vi "JKISM++ Example - Caller is NOT JKISM.vi"() -> ()   [LabVIEW 2014]
uses:
  user.lib/_NEVSTOP/JKI State Machine++/_Support/JKISMQ/_Create Data Queue.vi
  user.lib/_NEVSTOP/JKI State Machine++/_Support/JKISMQ/_JKISMQFGV.vi
  user.lib/_NEVSTOP/JKI State Machine++/JKI State Machine++.lvlib
panel:
  in  "UI: Front Panel State >> Close":bool
  in  "UI: Front Panel State >> Open":bool
  in  "API: Get Level":bool
  in  "Target Module":string(combo)="SubModule0"
  in  "Level":dbl min=0.0 max=1.0 step=0.1
  out "State History of Main":string
  in  "API: Stop":bool
  in  "API: Start":bool
  in  "Unregister Status Change":bool
  in  "Register Status Change":bool
  out "error":errorcluster
  in  "Stop Module":bool
  in  "Start Module":bool
  out "Exist?":bool
  # "Start/Stop Module"
  # "asdfasf"
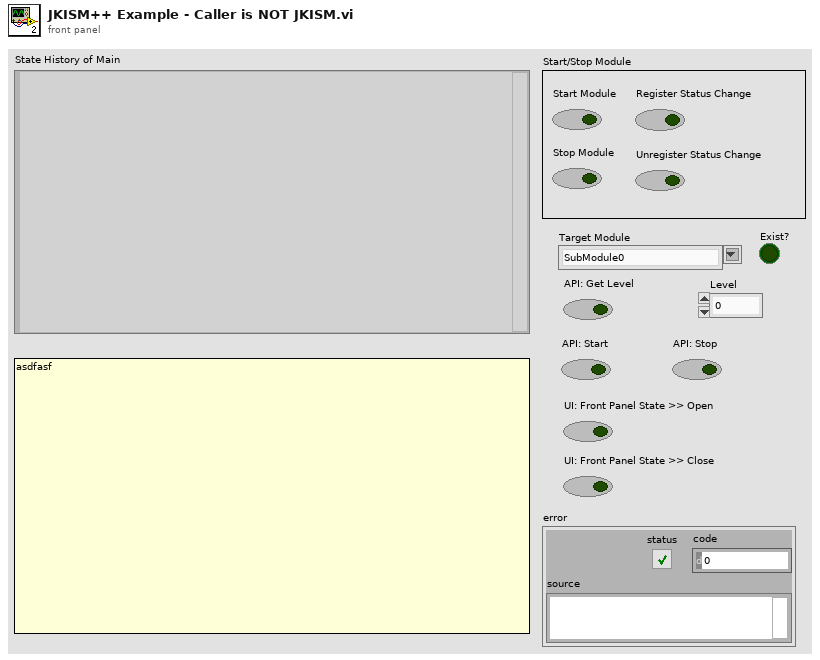
[diagram p1: front panel]
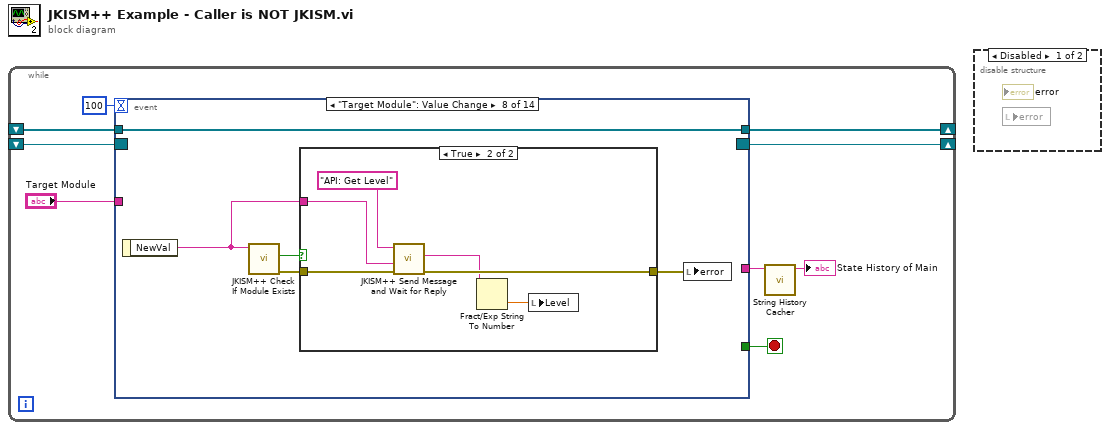
[diagram p0: block diagram]
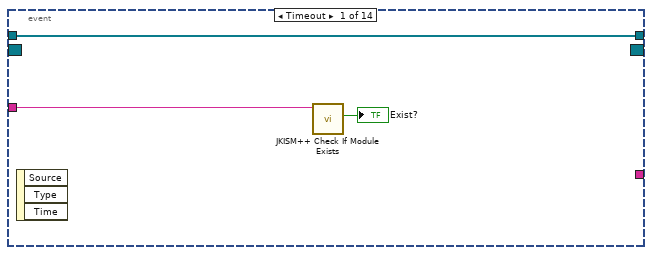
[diagram p3: hidden frame]
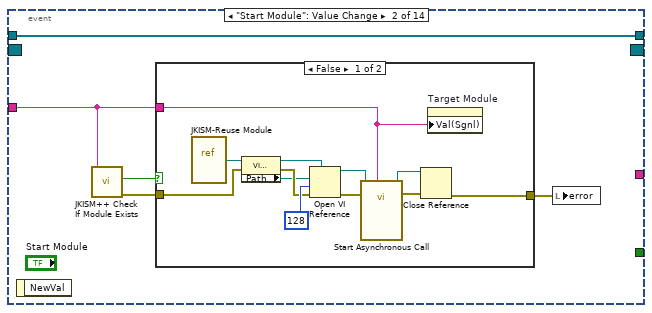
[diagram p4: hidden frame]
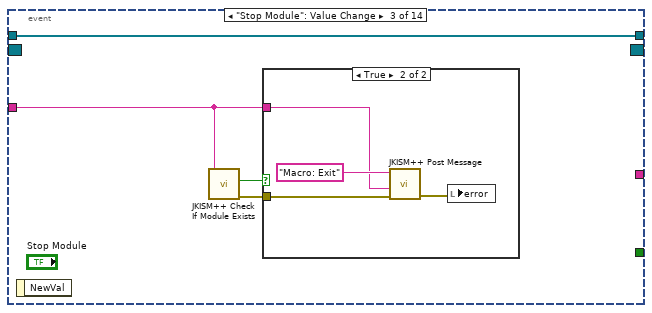
[diagram p6: hidden frame]
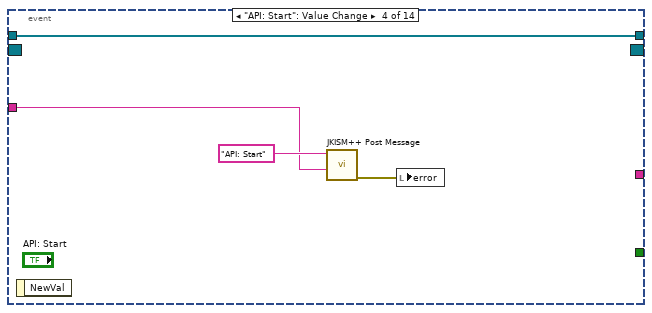
[diagram p8: hidden frame]
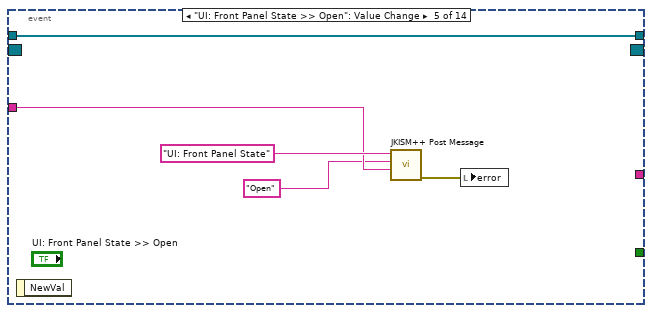
[diagram p9: hidden frame]
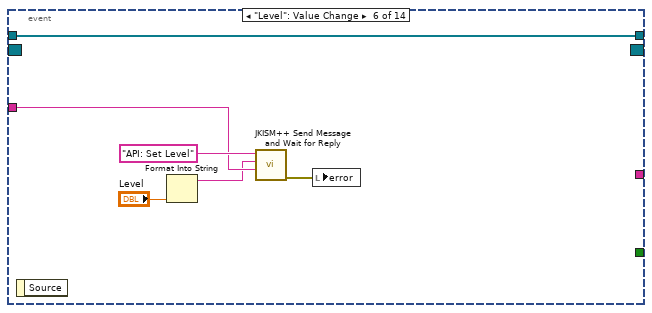
[diagram p10: hidden frame]
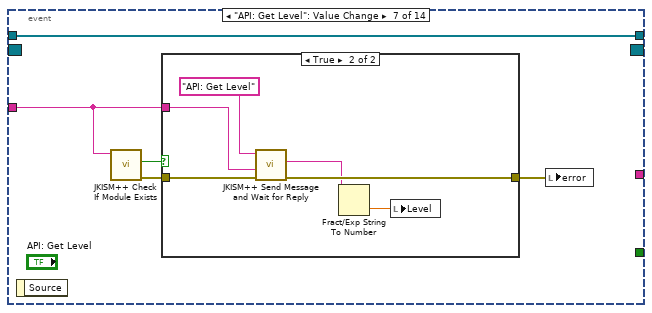
[diagram p11: hidden frame]
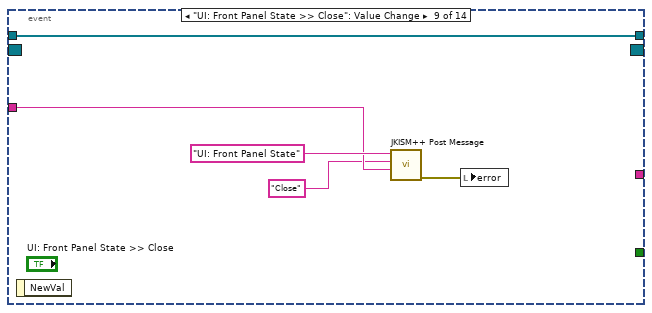
[diagram p14: hidden frame]
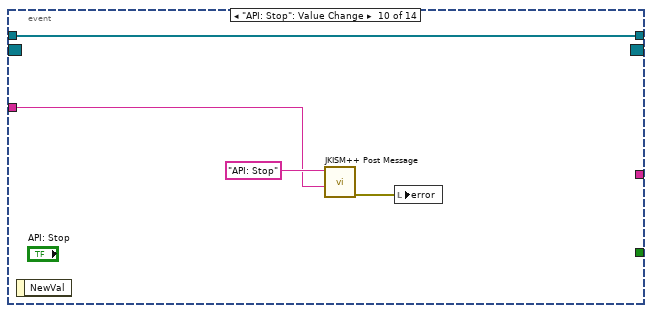
[diagram p15: hidden frame]
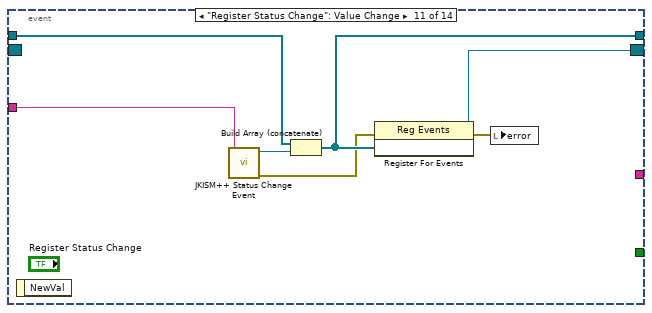
[diagram p16: hidden frame]
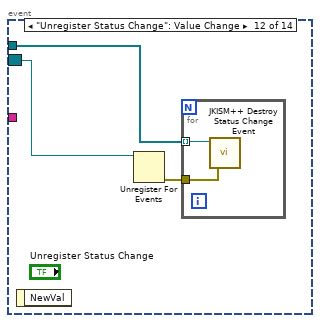
[diagram p17: hidden frame]
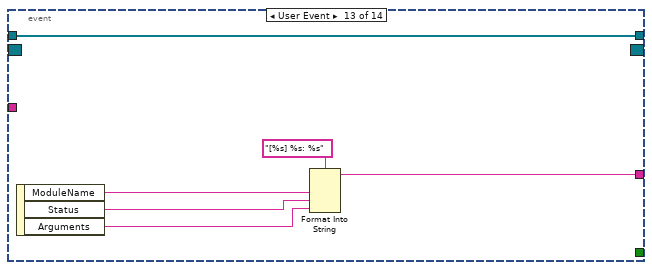
[diagram p18: hidden frame]
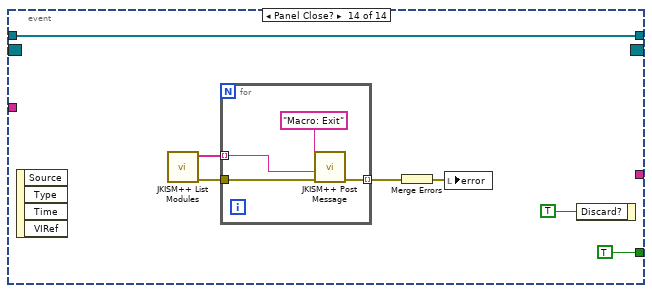
[diagram p19: hidden frame]
diagram:
  n1 = while {
    shift-right: [w7] -> _
    shift-left: _ -> [w6]
    shift-right: [w5] -> _
    shift-left: _ -> [w4]
    stop <- w9 stop-if-true
    n2 = event shown="[7] \"Target Module\": Value Change" {
      selector: w6 -> [_ _ _ _ _ _ _ _ _ _ _ w96 _ _]
      dyn-events: [_ _ _ _ _ _ _ _ _ _ w93 _ _ _] -> w7
      timeout: 100 -> [_ _ _ _ _ _ _ _ _ _ _ _ _ _]
      tunnel: [_ _ _ _ _ _ _ _ _ _ _ _ _ TRUE ("Discard?")] -> w9
      tunnel: [w12 w17 w34 w40 w45 w51 w57 w69 w80 w84 w92 _ w99 w109] -> w5
      tunnel: w4 -> [w12 w17 w34 w40 w45 w51 w57 w69 w80 w84 w90 w94 w99 w109]
      tunnel: [_ _ _ _ _ _ _ _ _ _ _ _ w100 _] -> w2
      tunnel: "Target Module" -> [w10 w13 w31 w39 w44 w50 w56 _ w79 w83 w89 _ _ _]
      event Timeout {
        n3 = event-data() -> ()  [unwired: 1 in, 3 out]
        n4 = call "JKISM++ Check If Module Exists.vi"("JKISM Name"=w10) -> ("Exist?"=→"Exist?":bool)  [unwired: 8 in, 2 out]
      }
      event "Start Module": Value Change {
        n5 = event-data() -> ()  [unwired: 1 in, 1 out]
        n6 = call "JKISM++ Check If Module Exists.vi"("JKISM Name"=w13) -> ("Error out"=w15:errorcluster, "Exist?"=w16:bool)  [unwired: 8 in, 1 out]
        n7 = case shown="False" w16 {
          tunnel: w15 -> [w20 w30]
          tunnel: [w19 w30] -> w14
          tunnel: w13 -> [w18 _]
          frame False {
            n8 = vi-ref "JKISM-Reuse Module.vi"() -> (w22:refnum<vi>)
            n9 = property class="VI (strict)"(reference=w22, error in=w20) -> (reference out=w26:refnum<vi>, error out=w24:errorcluster, "Path"=w23:path)
            n10 = Open VI Reference(type specifier VI Refnum (for type only)=w26, vi path=w23, options=128, error in (no error)=w24) -> (vi reference=w25:refnum<vi>, error out=w21:errorcluster)  [unwired: 2 in]
            n11 = call-by-ref "Start Asynchronous Call"(reference=w25, error in=w21, "Name(\"\" to use uuid)"=w18) -> (reference out=w28:refnum<vi>, error out=w27:errorcluster)  [unwired: 11 in]
            n12 = Close Reference(reference=w28, error in (no error)=w27) -> (error out=w19:errorcluster)
            n13 = property on="Target Module" class="CmbBox"("Val(Sgnl)"=w18) -> ()  [unwired: 2 in, 2 out]
          }
          frame True {
          }
        }
        n14 = local write "error"(w14) -> ()
      }
      event "Stop Module": Value Change {
        n15 = event-data() -> ()  [unwired: 1 in, 1 out]
        n16 = call "JKISM++ Check If Module Exists.vi"("JKISM Name"=w31) -> ("Error out"=w32:errorcluster, "Exist?"=w33:bool)  [unwired: 8 in, 1 out]
        n17 = case shown="True" w33 {
          tunnel: w32 -> [_ w36]
          tunnel: w31 -> [_ w35]
          frame False {
          }
          frame True {
            n18 = call "JKISM++ Post Message.vi"("Error In (no error)"=w36, "Target Module"=w35, "State"="Macro: Exit" ("States")) -> ("error out"=w37:errorcluster)  [unwired: 8 in]
            n19 = local write "error"(w37) -> ()
          }
        }
      }
      event "API: Start": Value Change {
        n20 = event-data() -> ()  [unwired: 1 in, 1 out]
        n21 = call "JKISM++ Post Message.vi"("Target Module"=w39, "State"="API: Start") -> ("error out"=w41:errorcluster)  [unwired: 9 in]
        n22 = local write "error"(w41) -> ()
      }
      event "UI: Front Panel State >> Open": Value Change {
        n23 = event-data() -> ()  [unwired: 1 in, 1 out]
        n24 = call "JKISM++ Post Message.vi"("Target Module"=w44, "Arguments (\"\")"="Open" ("Arguments (\"\")"), "State"="UI: Front Panel State") -> ("error out"=w46:errorcluster)  [unwired: 8 in]
        n25 = local write "error"(w46) -> ()
      }
      event "Level": Value Change {
        n26 = event-data() -> ()  [unwired: 1 in, 1 out]
        n27 = Format Into String("Level") -> (resulting string=w48:string)  [unwired: 3 in, 1 out]
        n28 = call "JKISM++ Send Message and Wait for Reply.vi"("Target Module"=w50, "Arguments (\"\")"=w48, "State"="API: Set Level") -> ("error out"=w52:errorcluster)  [unwired: 7 in, 1 out]
        n29 = local write "error"(w52) -> ()
      }
      event "API: Get Level": Value Change {
        n30 = event-data() -> ()  [unwired: 1 in, 1 out]
        n31 = call "JKISM++ Check If Module Exists.vi"("JKISM Name"=w56) -> ("Error out"=w55:errorcluster, "Exist?"=w54:bool)  [unwired: 8 in, 1 out]
        n32 = case shown="True" w54 {
          tunnel: [w59 w64] -> w58
          tunnel: w56 -> [_ w61]
          tunnel: w55 -> [w59 w60]
          frame False {
          }
          frame True {
            n33 = call "JKISM++ Send Message and Wait for Reply.vi"("Error In (no error)"=w60, "Target Module"=w61, "State"="API: Get Level") -> ("error out"=w64:errorcluster, "Arguments"=w62:string)  [unwired: 7 in]
            n34 = Fract/Exp String To Number(string=w62) -> (number=w63:dbl)  [unwired: 3 in, 1 out]
            n35 = local write "Level"(w63) -> ()
          }
        }
        n36 = local write "error"(w58) -> ()
      }
      event "Target Module": Value Change {
        n37 = event-data() -> ("NewVal"=w66:string)  [unwired: 1 in]
        n38 = call "JKISM++ Check If Module Exists.vi"("JKISM Name"=w66) -> ("Error out"=w68:errorcluster, "Exist?"=w67:bool)  [unwired: 8 in, 1 out]
        n39 = case shown="True" w67 {
          tunnel: [w71 w76] -> w70
          tunnel: w66 -> [_ w73]
          tunnel: w68 -> [w71 w72]
          frame False {
          }
          frame True {
            n40 = call "JKISM++ Send Message and Wait for Reply.vi"("Error In (no error)"=w72, "Target Module"=w73, "State"="API: Get Level") -> ("error out"=w76:errorcluster, "Arguments"=w74:string)  [unwired: 7 in]
            n41 = Fract/Exp String To Number(string=w74) -> (number=w75:dbl)  [unwired: 3 in, 1 out]
            n42 = local write "Level"(w75) -> ()
          }
        }
        n43 = local write "error"(w70) -> ()
      }
      event "UI: Front Panel State >> Close": Value Change {
        n44 = event-data() -> ()  [unwired: 1 in, 1 out]
        n45 = call "JKISM++ Post Message.vi"("Target Module"=w79, "Arguments (\"\")"="Close" ("Arguments (\"\")"), "State"="UI: Front Panel State") -> ("error out"=w81:errorcluster)  [unwired: 8 in]
        n46 = local write "error"(w81) -> ()
      }
      event "API: Stop": Value Change {
        n47 = event-data() -> ()  [unwired: 1 in, 1 out]
        n48 = call "JKISM++ Post Message.vi"("Target Module"=w83, "State"="API: Stop") -> ("error out"=w85:errorcluster)  [unwired: 9 in]
        n49 = local write "error"(w85) -> ()
      }
      event "Register Status Change": Value Change {
        n50 = event-data() -> ()  [unwired: 1 in, 1 out]
        n51 = call "JKISM++ Status Change Event.vi"("Name(\"\" to use uuid) in"=w89) -> ("Error out"=w88:errorcluster, "Status Change Event"=w91:refnum<user-event>)  [unwired: 9 in]
        n52 = Build Array (concatenate)(w90, w91) -> (w92:refnum<user-event>[])
        n53 = register-events(error in=w88, w92) -> (reference out=w93:refnum<event-registration>, error out=w87:errorcluster)  [unwired: 1 in]
        n54 = local write "error"(w87) -> ()
      }
      event "Unregister Status Change": Value Change {
        n55 = event-data() -> ()  [unwired: 1 in, 1 out]
        n56 = Unregister For Events(event registration refnum=w96) -> (error out=w95:errorcluster)  [unwired: 1 in]
        n57 = for {
          tunnel: w95 -> [w98]
          tunnel: w94 -> [w97] mode=indexing
          n58 = call "JKISM++ Destroy Status Change Event.vi"("Error in"=w98, "Status Change Event"=w97) -> ()  [unwired: 9 in, 1 out]
        }
      }
      event User Event {
        n59 = event-data() -> ("ModuleName"=w104:string, "Status"=w103:string, "Arguments"=w102:string)  [unwired: 1 in]
        n60 = Format Into String(format string="[%s] %s: %s", w104, w103, w102) -> (resulting string=w100:string)  [unwired: 2 in, 1 out]
      }
      event Panel Close? {
        n61 = event-data() -> ()  [unwired: 1 in, 4 out]
        n62 = call "JKISM++ List Modules.vi"() -> ("Error out"=w106:errorcluster, "Module Names"=w105:string[])  [unwired: 10 in]
        n63 = for {
          tunnel: [w114] -> w108 mode=indexing
          tunnel: w106 -> [w113]
          tunnel: w105 -> [w112] mode=indexing
          n64 = call "JKISM++ Post Message.vi"("Error In (no error)"=w113, "Target Module"=w112, "State"="Macro: Exit" ("States")) -> ("error out"=w114:errorcluster)  [unwired: 8 in]
        }
        n65 = Merge Errors(w108) -> (w107:errorcluster)
        n66 = local write "error"(w107) -> ()
        n67 = event-data("Discard?"=TRUE) -> ()  [unwired: 1 in, 1 out]
      }
    }
    n68 = call "String History Cacher.vi"("String"=w2) -> ("String Cache"=→"State History of Main":string)  [unwired: 10 in]
  }
  n69 = disable-structure shown="Disabled" {
    frame Disabled {
      n70 = local read "error"() -> ()  [unwired: 1 in]
    }
    frame Enabled {
    }
  }
